vi "Scale_Plot.vi"(0 "Cluster":cluster{"Y":dbl[], "X":dbl[]}, 1 "Boolesch":bool=TRUE, 2 "Scale 1":dbl) -> (5 "Cluster 2":cluster{"Y":dbl[], "X":dbl[]})   [LabVIEW 2016]
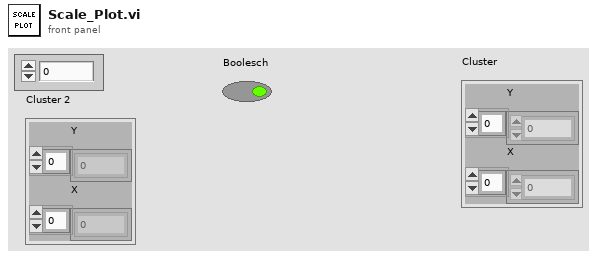
[diagram p1: front panel]
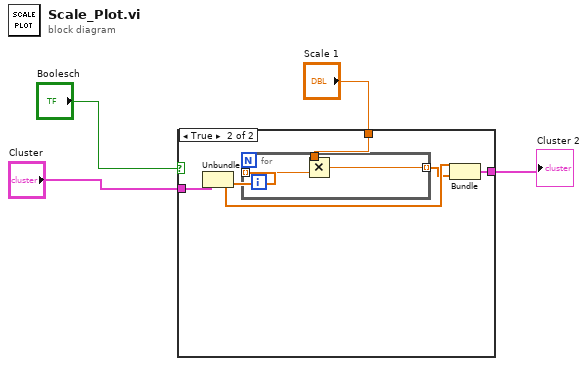
[diagram p0: block diagram]
diagram:
  n1 = case shown="True" "Boolesch" {
    tunnel: "Scale 1" -> [_ w11]
    tunnel: [w5 w10] -> w1
    tunnel: "Cluster" -> [w5 w9]
    frame False {
    }
    frame True {
      n2 = Unbundle(w9) -> ("Y"=w7:dbl[], "X"=w8:dbl[])
      n3 = for {
        tunnel: w8 -> [w14] mode=indexing
        tunnel: w11 -> [w13]
        tunnel: [w12] -> w6 mode=indexing
        n4 = Multiply(x=w13, y=w14) -> (x*y=w12:dbl)
      }
      n5 = Bundle("Y"=w7, w6) -> (w10:cluster{"Y":dbl[], dbl[]})  [unwired: 1 in]
    }
  }
  "Cluster 2" <- w1
